vi "writeData.vi"(0 "base path":path, 1 "time stamp":timestamp, 2 "Parameters":string[](array[string]), 3 "error in":errorcluster, 4 "Input data":waveform(dbl)[](array[waveform])) -> (7 "error out":errorcluster)   [LabVIEW 2023]
uses:
  <vilib>/Utility/file.llb/Write Delimited Spreadsheet (string).vi
  <vilib>/Waveform/WDTOps.llb/WDT Index Channel DBL.vi
  <vilib>/Utility/file.llb/Write Delimited Spreadsheet (DBL).vi
panel:
  out "Waveform Graph":waveform(dbl)[](graph)
  in  "time format string (%c)":string="mmddYYYY_HHMMSS"
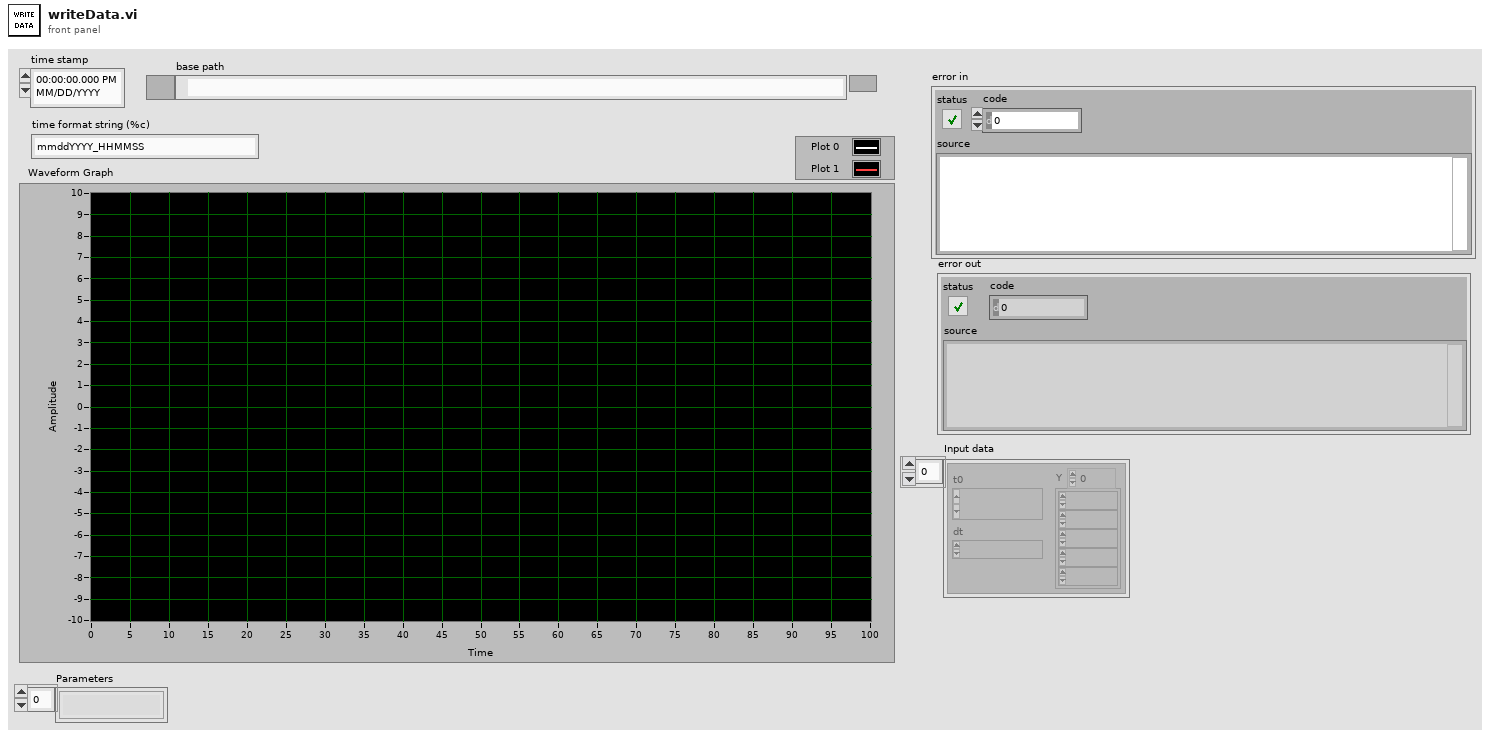
[diagram p1: front panel]
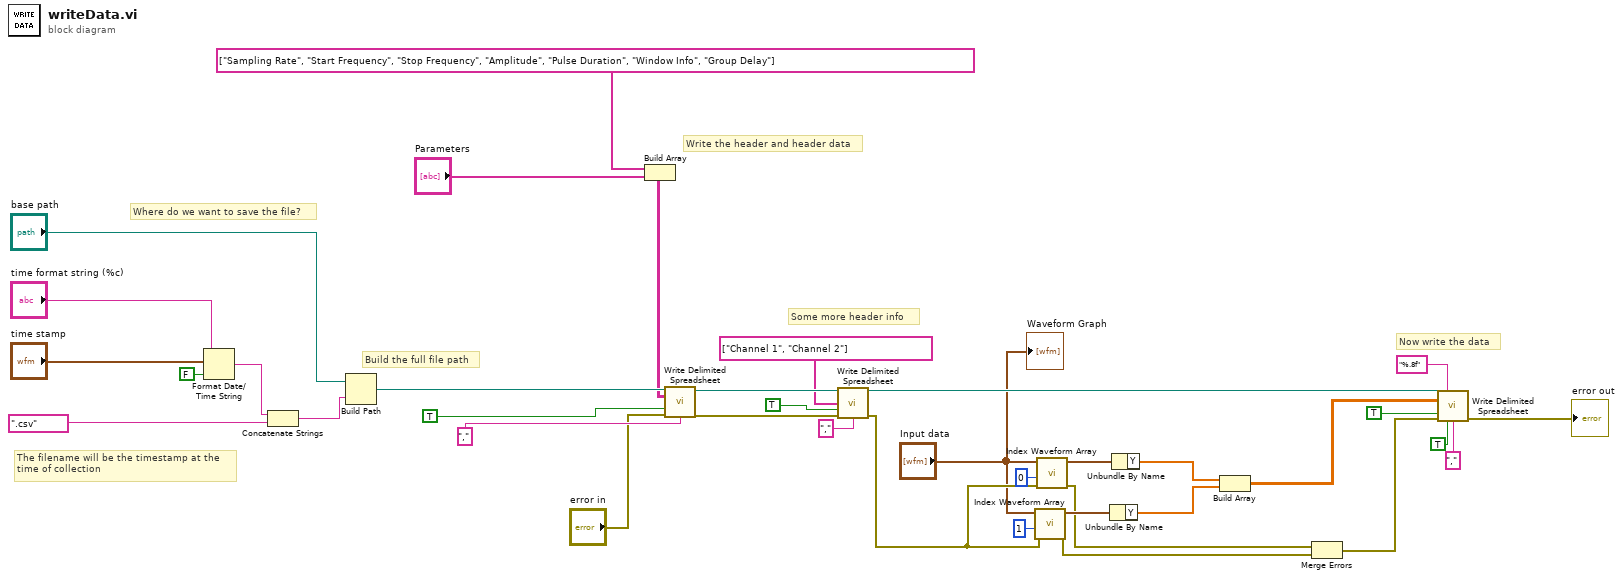
[diagram p0: block diagram]
diagram:
  # "Now write the data"
  # "Some more header info"
  # "Write the header and header data"
  # "Build the full file path"
  # "The filename will be the timestamp at the\ntime of collection"
  # "Where do we want to save the file?"
  n1 = Format Date/Time String(time format string (%c)="time format string (%c)", seconds (now)="time stamp", UTC format=FALSE) -> (date/time string=w36:string)
  n2 = Concatenate Strings(w36, ".csv" ("string")) -> (w35:string)
  n3 = Build Path(base path="base path", name or relative path=w35) -> (appended path=w18:path)
  n4 = Build Array(string[] ["Sampling Rate", "Start Frequency", "Stop Frequency", "Amplitude", "Pulse Duration", "Window Info", "Group Delay"], "Parameters") -> (w13:string[][])
  n5 = call-poly <vilib>:"Write Delimited Spreadsheet.vi"("file path (dialog if empty)"=w18, "2D data"=w13, "append to file? (new file:F)"=TRUE, "error in (no error)"="error in", "delimiter (\\t)"="," ("delimiter (\\t)")) -> ("new file path (Not A Path if cancelled)"=w15:path, "error out"=w14:errorcluster)  [unwired: 9 in]
  n6 = call-poly <vilib>:"Write Delimited Spreadsheet.vi"("file path (dialog if empty)"=w15, "1D data"=string[] ["Channel 1", "Channel 2"], "append to file? (new file:F)"=TRUE, "error in (no error)"=w14, "delimiter (\\t)"="," ("delimiter (\\t)")) -> ("new file path (Not A Path if cancelled)"=w10:path, "error out"=w11:errorcluster)  [unwired: 9 in]
  n7 = call-poly <vilib>:"Index Waveform Array.vi"("error in (no error)"=w11, "index"=1, "waveform array"="Input data") -> ("error out"=w19:errorcluster, "waveform"=w25:waveform(dbl))  [unwired: 7 in]
  n8 = call-poly <vilib>:"Index Waveform Array.vi"("error in (no error)"=w11, "index"=0, "waveform array"="Input data") -> ("error out"=w20:errorcluster, "waveform"=w27:waveform(dbl))  [unwired: 7 in]
  n9 = Unbundle By Name(w25) -> ("Y"=w22:dbl[])
  n10 = Unbundle By Name(w27) -> ("Y"=w26:dbl[])
  n11 = Build Array(w26, w22) -> (w7:dbl[][])
  n12 = Merge Errors(w20, w19) -> (w21:errorcluster)
  n13 = call-poly <vilib>:"Write Delimited Spreadsheet.vi"("file path (dialog if empty)"=w10, "format (%.3f)"="%.8f", "2D data"=w7, "append to file? (new file:F)"=TRUE, "error in (no error)"=w21, "transpose? (no:F)"=TRUE, "delimiter (\\t)"="," ("delimiter (\\t)")) -> ("error out"=→"error out":errorcluster)  [unwired: 7 in, 1 out]
  "Waveform Graph" <- "Input data"
